vi "solar Create (LVClass.ini).vi"(8 "error in (no error)":errorcluster, 11 "Default LVClass":refnum<class "solar.lvclass">) -> (0 "error out":errorcluster, 2 "LVClass":string, 3 "solar out":refnum<class "solar.lvclass">)   [LabVIEW 2018, in "solar.lvclass"]
doc: "This loads the target's 'LVClass' configuration item. The 'LVClass' key determines whitch SOLAR target class to inherit from."
uses:
  solar.lvclass
  cfg/solar_cfg Read File (Str).vi
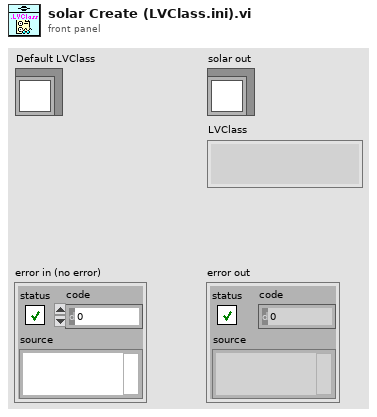
[diagram p1: front panel]
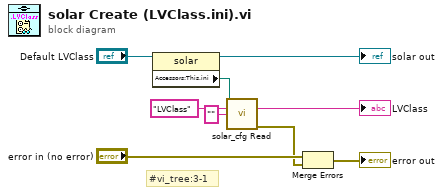
[diagram p0: block diagram]
diagram:
  # "#vi_tree:3-1"
  n1 = property class="solar"(reference="Default LVClass") -> (reference out=→"solar out":refnum<class "solar.lvclass">, "Accessors:This.ini"=w8:path)  [unwired: 1 in, 1 out]
  n2 = call-poly "solar_cfg Read.vi"("Config Path (*.ini)"=w8, "Key"="LVClass" ("Key_Prefix (\"\")"), "Value in"="") -> ("Value out"=→"LVClass":string, "error out"=w2:errorcluster)  [unwired: 9 in, 2 out]
  n3 = Merge Errors("error in (no error)", w2) -> (→"error out":errorcluster)
